vi "add_range_AC_check_to_report.vi"(8 "error in (no error)":errorcluster, 11 "Boc12 in":refnum<class "Boc12.lvclass">) -> (0 "error out":errorcluster, 3 "Boc12 out":refnum<class "Boc12.lvclass">)   [LabVIEW 2017, in "Boc12.lvclass"]
uses:
  Boc12.lvclass
  Report.lvclass/Report.ctl
  <vilib>/Utility/NIReport.llb/Append Text Table to Report (wrap).vi
  <vilib>/Utility/NIReport.llb/NI_report.lvclass
  Report.lvclass
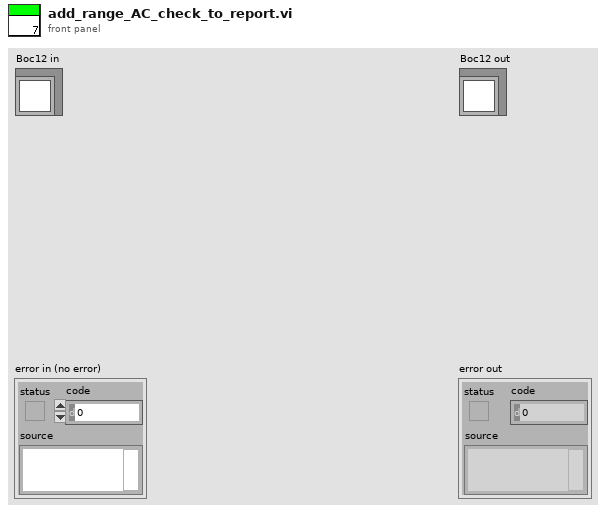
[diagram p1: front panel]
types:
  T1 = cluster{"position (excel)":cluster{"row":i32, "column":i32}, "name (excel)":string, "bookmark (word)":string}
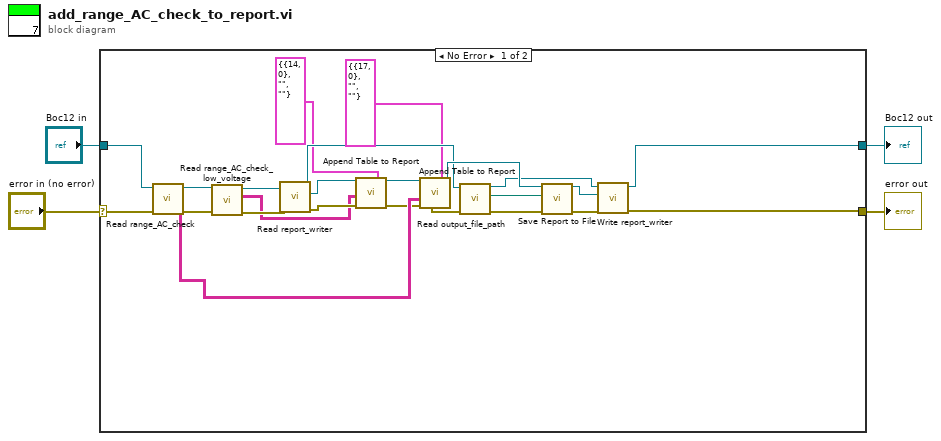
[diagram p0: block diagram]
diagram:
  n1 = case shown="No Error" "error in (no error)" {
    selector: "error in (no error)" -> [w27 w29]
    tunnel: "Boc12 in" -> [w28 w30]
    tunnel: [w15 w30] -> w3
    tunnel: [w16 w29] -> w2
    frame No Error {
      n2 = call-dynamic "Read range_AC_check.vi"("error in (no error)"=w27, "Report in"=w28) -> ("error out"=w12:errorcluster, "range_AC_check"=w18:string[][], "Report out"=w14:refnum<class "Boc12.lvclass">)  [unwired: 7 in]
      n3 = call-dynamic "Read range_AC_check_low_voltage.vi"("error in (no error)"=w12, "Report in"=w14) -> ("error out"=w11:errorcluster, "range_AC_check_low_voltage"=w6:string[][], "Report out"=w13:refnum<class "Boc12.lvclass">)  [unwired: 7 in]
      n4 = call "Read report_writer.vi"("error in (no error)"=w11, "Report in"=w13) -> ("error out"=w7:errorcluster, "NI_report.lvclass"=w8:refnum<class "NI_report.lvclass">, "Report out"=w23:refnum<class "Boc12.lvclass">)  [unwired: 7 in]
      n5 = call-poly <vilib>:"Append Table to Report.vi"("report in"=w8, "MS Office parameters"=T1 {"position (excel)"={"row"=14, "column"=0}, "name (excel)"="", "bookmark (word)"=""}, "text data"=w6, "error in (no error)"=w7) -> ("report out"=w9:refnum<class "NI_report.lvclass">, "error out"=w10:errorcluster)  [unwired: 8 in, 2 out]
      n6 = call-poly <vilib>:"Append Table to Report.vi"("report in"=w9, "MS Office parameters"=T1 {"position (excel)"={"row"=17, "column"=0}, "name (excel)"="", "bookmark (word)"=""}, "text data"=w18, "error in (no error)"=w10) -> ("report out"=w26:refnum<class "NI_report.lvclass">, "error out"=w24:errorcluster)  [unwired: 8 in, 2 out]
      n7 = call "Read output_file_path.vi"("error in (no error)"=w24, "Report in"=w23) -> ("error out"=w25:errorcluster, "output_file_path"=w19:path, "Report out"=w20:refnum<class "Boc12.lvclass">)  [unwired: 7 in]
      n8 = call-dynamic "Save Report to File.vi"("report in"=w26, "report file path"=w19, "error in (no error)"=w25) -> ("report out"=w21:refnum<class "NI_report.lvclass">, "error out"=w22:errorcluster)  [unwired: 11 in]
      n9 = call "Write report_writer.vi"("error in (no error)"=w22, "NI_report.lvclass"=w21, "Report in"=w20) -> ("error out"=w16:errorcluster, "Report out"=w15:refnum<class "Boc12.lvclass">)  [unwired: 7 in]
    }
    frame Error {
    }
  }
  "error out" <- w2
  "Boc12 out" <- w3
